vi "FringeTracker-Optimize.vi"() -> ()   [LabVIEW 2009]
uses:
  <vilib>/Analysis/Matrix/Datatypes/RealMatrix.ctl
  <vilib>/Analysis/baseanly.llb/A x Vector.vi
  <vilib>/Analysis/baseanly.llb/Real A x B.vi
  <vilib>/Analysis/Matrix/Numeric/Conversions/Array To Matrix - RA2.vi
  Instruments/RTC/Api/TelemetryServer/TelemetryServer_Global.vi
  <vilib>/Analysis/NI_AALBase.lvlib
  <vilib>/Analysis/Matrix/NI_Matrix.lvlib
panel:
  in  "stop":bool
  in  "Telescopes":i32(ring) items=["K1", "K2"]
  in  "ALIGN Button":bool
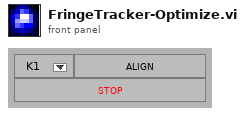
[diagram p1: front panel]
types:
  T1 = typedef "NI_Matrix.lvlib/RealMatrix.ctl" = dbl[][]
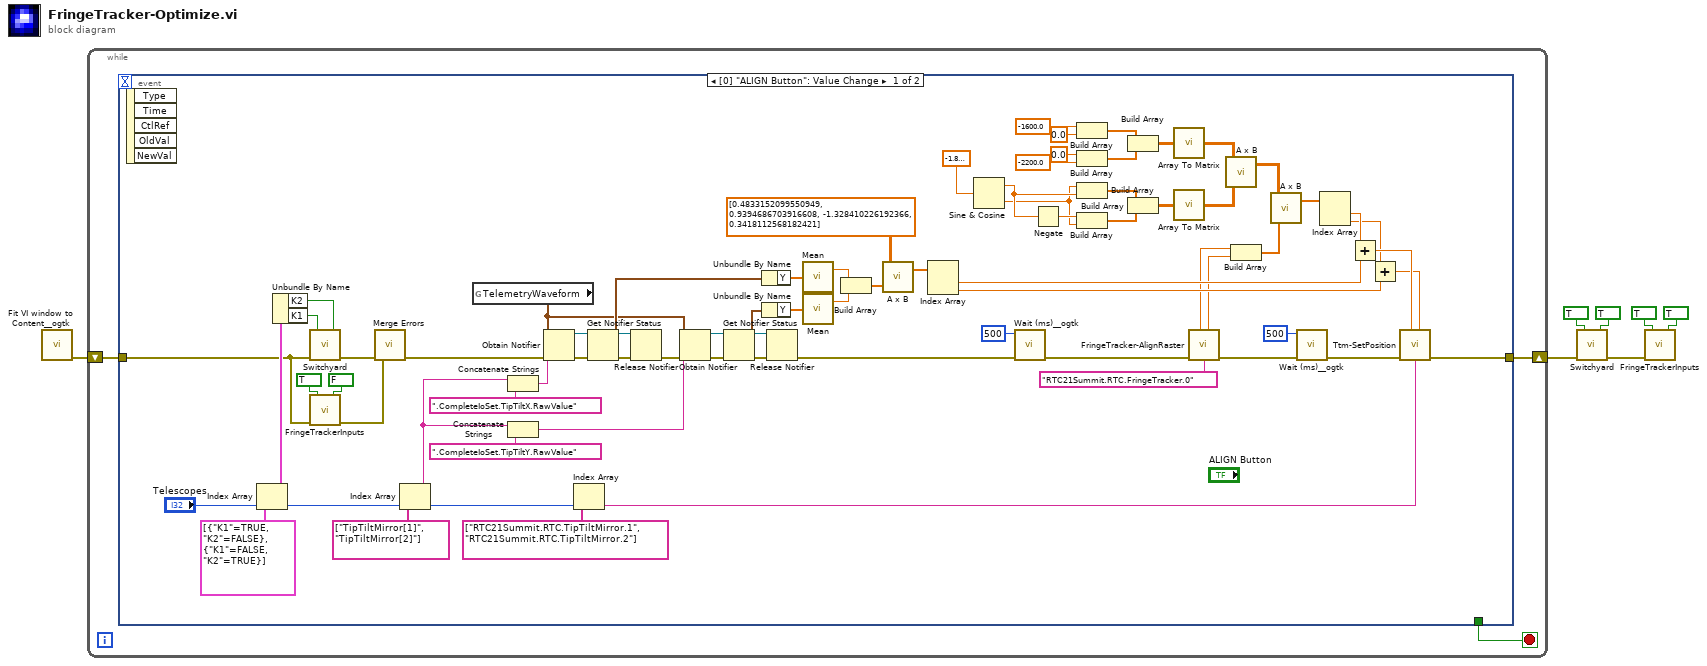
[diagram p0: block diagram]
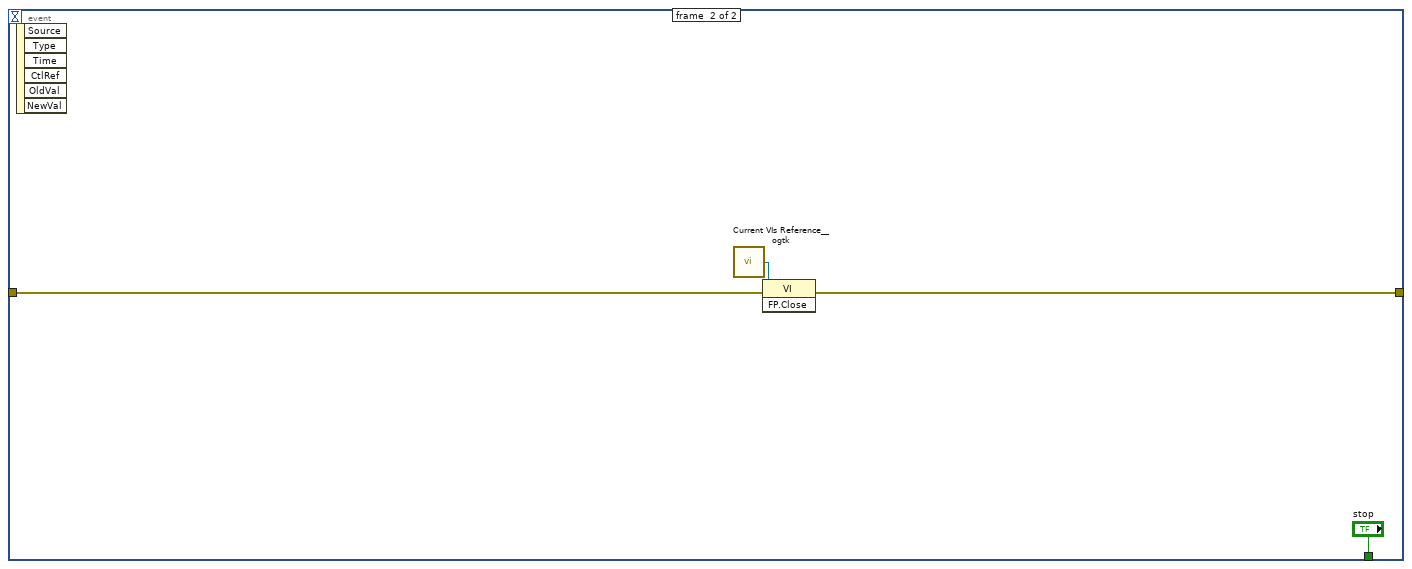
[diagram p2: hidden frame]
diagram:
  n1 = call <userlib>:"Fit VI window to Content__ogtk.vi"() -> ("error out"=w4:errorcluster)  [unwired: 3 in, 4 out]
  n2 = while {
    shift-right: [w10] -> w7
    shift-left: w4 -> [w9]
    stop <- w8 stop-if-true
    n3 = event shown="[0] \"ALIGN Button\": Value Change" {
      selector: _ -> [_ _]
      dyn-events: _ -> [_ _]
      timeout: _ -> [_ _]
      tunnel: [w19 w84] -> w10
      tunnel: w9 -> [w14 w85]
      tunnel: [_ "stop"] -> w8
      event #0 {
        n4 = event-data() -> ()  [unwired: 6 out]
        n5 = Index Array(array=cluster{"K1":bool, "K2":bool}[] [{"K1"=TRUE, "K2"=FALSE}, {"K1"=FALSE, "K2"=TRUE}], index="Telescopes") -> (element=w50:cluster{"K1":bool, "K2":bool})
        n6 = Unbundle By Name(w50) -> ("K2"=w48:bool, "K1"=w49:bool)
        n7 = call "Switchyard.vi"("K2"=w48, "K1"=w49, "error in (no error)"=w14) -> ("error out"=w13:errorcluster)  [unwired: 4 out]
        n8 = call "FringeTrackerInputs.vi"("SPEC"=FALSE, "WL"=TRUE, "error in (no error)"=w14) -> ("error out"=w12:errorcluster)  [unwired: 4 out]
        n9 = call <vilib>:"Merge Errors.vi"("error in 3 (no error)"=w12, "error in 2 (no error)"=w13) -> ("error out"=w11:errorcluster)  [unwired: 2 in, 3 out]
        n10 = Index Array(array=string[] ["TipTiltMirror[1]", "TipTiltMirror[2]"], index="Telescopes") -> (element=w55:string)
        n11 = global read "TelemetryServer_Global.vi" "TelemetryWaveform"() -> (w53:waveform(dbl))
        n12 = Concatenate Strings(w55, ".CompleteIoSet.TipTiltX.RawValue" ("Telemetry")) -> (w57:string)
        n13 = Concatenate Strings(w55, ".CompleteIoSet.TipTiltY.RawValue" ("Telemetry")) -> (w54:string)
        n14 = Obtain Notifier(name (unnamed)=w57, notification data type=w53, error in (no error)=w11) -> (notifier out=w80:refnum<notifier>, error out=w81:errorcluster)  [unwired: 1 in, 1 out]
        n15 = Index Array(array=string[] ["RTC21Summit.RTC.TipTiltMirror.1", "RTC21Summit.RTC.TipTiltMirror.2"], index="Telescopes") -> (element=w18:string)
        n16 = Get Notifier Status(notifier=w80, error in (no error)=w81) -> (notifier out=w76:refnum<notifier>, current notification=w72:waveform(dbl), error out=w77:errorcluster)  [unwired: 2 out]
        n17 = Release Notifier(notifier=w76, error in (no error)=w77) -> (error out=w73:errorcluster)  [unwired: 3 out]
        n18 = Obtain Notifier(name (unnamed)=w54, notification data type=w53, error in (no error)=w73) -> (notifier out=w79:refnum<notifier>, error out=w78:errorcluster)  [unwired: 1 in, 1 out]
        n19 = Get Notifier Status(notifier=w79, error in (no error)=w78) -> (notifier out=w75:refnum<notifier>, current notification=w71:waveform(dbl), error out=w74:errorcluster)  [unwired: 2 out]
        n20 = Unbundle By Name(w72) -> ("Y"=w70:dbl[])
        n21 = Unbundle By Name(w71) -> ("Y"=w69:dbl[])
        n22 = Release Notifier(notifier=w75, error in (no error)=w74) -> (error out=w68:errorcluster)  [unwired: 3 out]
        n23 = call <vilib>:"Mean.vi"("X"=w70) -> ("mean"=w67:dbl)  [unwired: 1 out]
        n24 = call <vilib>:"Mean.vi"("X"=w69) -> ("mean"=w66:dbl)  [unwired: 1 out]
        n25 = Build Array(w67, w66) -> (w65:dbl[])
        n26 = call-poly <vilib>:"A x B.vi"("Vector"=w65, "A"=T1 [[0.4833152099550949, 0.9394686703916608], [-1.328410226192366, 0.3418112568182421]] ("Inverse Matrix")) -> ("A x Vector"=w64:dbl[])  [unwired: 1 out]
        n27 = Index Array(array=w64) -> (element #1=w62:dbl, element #2=w61:dbl)  [unwired: 2 in]
        n28 = Sine & Cosine(0:dbl[unit] -1.8675022996339325 ("Angle")) -> (1:w40:dbl, 2:w38:dbl)
        n29 = call <userlib>:"Wait (ms)__ogtk.vi"("error in (no error)"=w68, "milliseconds to wait"=u32 500) -> ("error out"=w82:errorcluster)  [unwired: 1 in, 8 out]
        n30 = Negate(x=w40) -> (-x=w39:dbl)
        n31 = Build Array(-1600.0 ("Echelle"), 0.0 ("element")) -> (w35:dbl[])
        n32 = Build Array(0.0 ("element"), -2200.0 ("Echelle 2")) -> (w36:dbl[])
        n33 = Build Array(w38, w40) -> (w42:dbl[])
        n34 = Build Array(w39, w38) -> (w41:dbl[])
        n35 = Build Array(w35, w36) -> (w31:dbl[][])
        n36 = Build Array(w42, w41) -> (w37:dbl[][])
        n37 = call-poly <vilib>:"Array To Matrix.vi"("Real 2D Array"=w31) -> ("Real Matrix"=w29:T1)
        n38 = call-poly <vilib>:"Array To Matrix.vi"("Real 2D Array"=w37) -> ("Real Matrix"=w28:T1)
        n39 = call "FringeTracker-AlignRaster.vi"("error in (no error)"=w82, "FringeTracker name"="RTC21Summit.RTC.FringeTracker.0") -> ("error out"=w23:errorcluster, "xOffset"=w44:dbl, "yOffset"=w43:dbl)  [unwired: 6 out]
        n40 = call-poly <vilib>:"A x B.vi"("B"=w28, "A"=w29) -> ("A x B"=w27:T1)  [unwired: 1 out]
        n41 = Build Array(w44, w43) -> (w26:dbl[])
        n42 = call-poly <vilib>:"A x B.vi"("Vector"=w26, "A"=w27) -> ("A x Vector"=w17:dbl[])  [unwired: 1 out]
        n43 = call <userlib>:"Wait (ms)__ogtk.vi"("error in (no error)"=w23, "milliseconds to wait"=u32 500) -> ("error out"=w22:errorcluster)  [unwired: 1 in, 8 out]
        n44 = Index Array(array=w17) -> (element #1=w25:dbl, element #2=w24:dbl)  [unwired: 2 in]
        n45 = Add(x=w25, y=w62) -> (x+y=w47:dbl)
        n46 = Add(x=w24, y=w61) -> (x+y=w46:dbl)
        n47 = call "Ttm-SetPosition.vi"("error in (no error)"=w22, "Ttm Name"=w18, "X"=w47, "Y"=w46) -> ("error out"=w19:errorcluster)  [unwired: 6 out]
      }
      event #1 {
        n48 = event-data() -> ()  [unwired: 7 out]
        n49 = call <userlib>:"Current VIs Reference__ogtk.vi"() -> ("Current VI's reference"=w86:refnum<vi>)  [unwired: 5 out]
        n50 = invoke class="VI" method="FP.Close"(reference=w86, error in=w85) -> (error out=w84:errorcluster)  [unwired: 1 in, 2 out]
      }
    }
  }
  n51 = call "Switchyard.vi"("K2"=TRUE, "K1"=TRUE, "error in (no error)"=w7) -> ("error out"=w1:errorcluster)  [unwired: 4 out]
  n52 = call "FringeTrackerInputs.vi"("SPEC"=TRUE, "WL"=TRUE, "error in (no error)"=w1) -> ()  [unwired: 5 out]
